vi "OAT Unfiltered Orbit Plot.vi"   [LabVIEW 2017]
doc: "Draws an orbit plot of waveform signals on a XY graph. You can use sampled or resampled waveform signals from proximity transducers. You can use this polymorphic VI to draw an orbit plot of resampled signals or waveform signals. The data types you wire to the <B>resampled signal(X)</B> and <B>resampled signal (Y)</B> inputs determine the polymorphic instance to use."
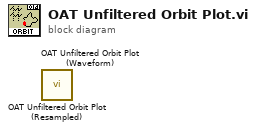
[diagram p0: block diagram]
diagram:
  n1 = call <vilib>:"OAT Unfiltered Orbit Plot (Resampled).vi"() -> ()  [unwired: 14 in, 2 out]
  n2 = call <vilib>:"OAT Unfiltered Orbit Plot (Waveform).vi"() -> ()  [unwired: 14 in, 2 out]
